vi "Example.vi"   [LabVIEW 2013]
uses:
  T560TriggerClass/T560Trigger.lvclass
  T560SessionClass/T560Session.lvclass
  Common/TypeDefs/TriggerImpedance.ctl
  Common/TypeDefs/ChannelPolarity.ctl
  Common/TypeDefs/TriggerSource.ctl
  T560OutputClass/T560Output.lvclass
  Common/TypeDefs/ChannelName.ctl
  T560ChannelClass/T560Channel.lvclass
types:
  T1 = typedef "T560Channel.lvclass/ChannelName.ctl" = enum16{"Null", "A", "B", "C", "D", "Trigger"}
  T2 = typedef "TriggerSource.ctl" = enum16{"Rising", "Falling", "Internal 80MHz", "Internal DDS", "Remote", "Disabled"}
  T3 = typedef "ChannelPolarity.ctl" = enum16{"Direct", "Inverted"}
  T4 = typedef "TriggerImpedance.ctl" = enum16{"10KOhm", "50Ohms"}
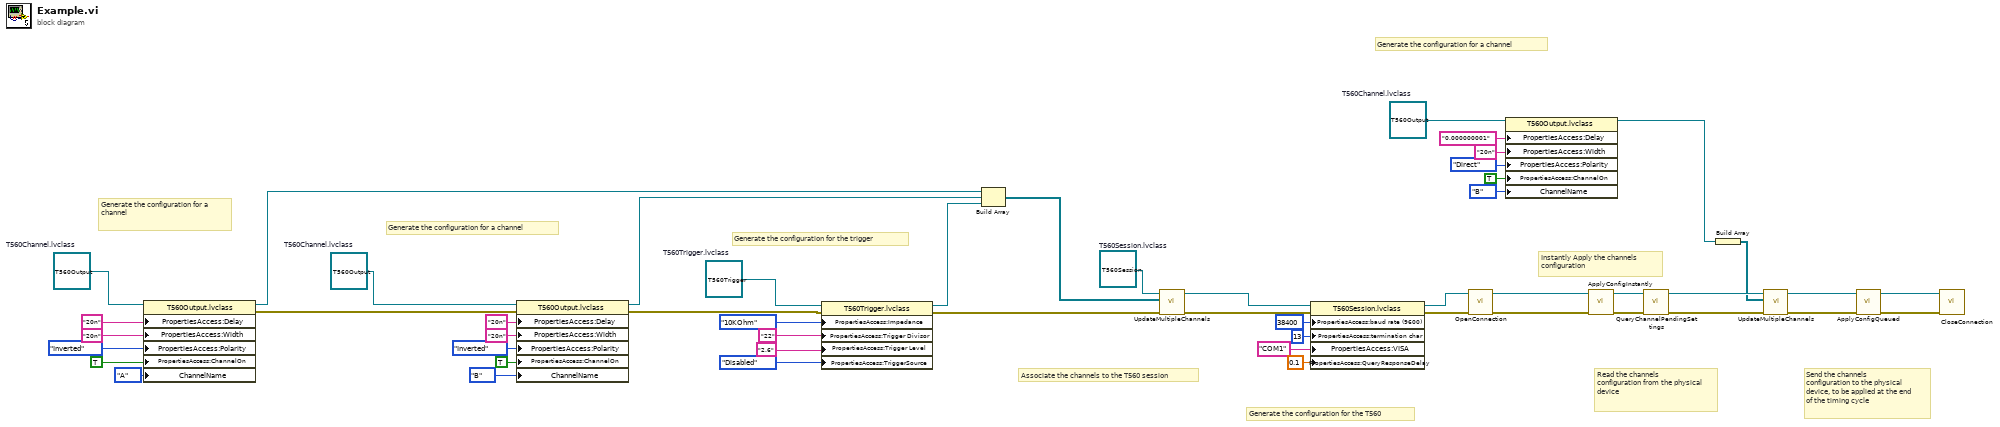
[diagram p0: block diagram]
diagram:
  w21 = refnum<class "T560Output.lvclass"> refnum  # T560Channel.lvclass
  w20 = refnum<class "T560Output.lvclass"> refnum  # T560Channel.lvclass
  w16 = refnum<class "T560Output.lvclass"> refnum  # T560Channel.lvclass
  w10 = refnum<class "T560Session.lvclass"> refnum  # T560Session.lvclass
  w51 = refnum<class "T560Trigger.lvclass"> refnum  # T560Trigger.lvclass
  # "Read the channels configuration from the physical device"
  # "Send the channels configuration to the physical device, to be applied at the end of the timing cycle"
  # "Generate the configuration for a channel"
  # "Instantly Apply the channels \nconfiguration"
  # "Generate the configuration for the T560"
  # "Associate the channels to the T560 session"
  # "Generate the configuration for a channel"
  # "Generate the configuration for the trigger"
  # "Generate the configuration for a channel"
  n1 = property class="T560Output.lvclass"(reference=w16, "PropertiesAccess:Delay"="20n" ("Delay"), "PropertiesAccess:Width"="20n" ("Width"), "PropertiesAccess:Polarity"=ChannelPolarity."Inverted" ("Polarity"), "PropertiesAccess:ChannelOn"=TRUE ("ChannelOn"), "ChannelName"=ChannelName."A") -> (reference out=w36:refnum<class "T560Output.lvclass">, error out=w19:errorcluster)  [unwired: 1 in]
  n2 = property class="T560Output.lvclass"(reference=w20, error in=w19, "PropertiesAccess:Delay"="20n" ("Delay"), "PropertiesAccess:Width"="20n" ("Width"), "PropertiesAccess:Polarity"=ChannelPolarity."Inverted" ("Polarity"), "PropertiesAccess:ChannelOn"=TRUE ("ChannelOn"), "ChannelName"=ChannelName."B") -> (reference out=w35:refnum<class "T560Output.lvclass">, error out=w34:errorcluster)
  n3 = property class="T560Trigger.lvclass"(reference=w51, error in=w34, "PropertiesAccess:Impedance"=TriggerImpedance."10KOhm" ("Impedance"), "PropertiesAccess:Trigger Divisor"="22" ("Trigger Divisor"), "PropertiesAccess:Trigger Level"="2.6" ("Trigger Divisor"), "PropertiesAccess:TriggerSource"=TriggerSource."Disabled" ("TriggerSource")) -> (reference out=w41:refnum<class "T560Trigger.lvclass">, error out=w11:errorcluster)
  n4 = Build Array(w36, w35, w41) -> (w8:refnum<class "T560Channel.lvclass">[])
  n5 = call-dynamic "UpdateMultipleChannels.vi"("error in (no error)"=w11, "ChannelsIn"=w8, "T560Session in"=w10) -> ("error out"=w7:errorcluster, "T560Session out"=w9:refnum<class "T560Session.lvclass">)  [unwired: 7 in]
  n6 = property class="T560Session.lvclass"(reference=w9, error in=w7, "PropertiesAccess:baud rate (9600)"=u32 38400 ("baud rate (9600)"), "PropertiesAccess:termination char"=u8 13 ("termination char"), "PropertiesAccess:VISA"="COM1" ("VISA"), "PropertiesAccess:QueryResponseDelay"=0.1 ("QueryResponseDelay")) -> (reference out=w32:refnum<class "T560Session.lvclass">, error out=w33:errorcluster)
  n7 = call-dynamic "OpenConnection.vi"("error in"=w33, "T560Session in"=w32) -> ("error out"=w43:errorcluster, "T560Session out"=w42:refnum<class "T560Session.lvclass">)  [unwired: 8 in]
  n8 = property class="T560Output.lvclass"(reference=w21, "PropertiesAccess:Delay"="0.000000001" ("Delay"), "PropertiesAccess:Width"="20n" ("Width"), "PropertiesAccess:Polarity"=enum16{"Direct", "Inverted"}."Direct" ("Polarity"), "PropertiesAccess:ChannelOn"=TRUE ("ChannelOn"), "ChannelName"=ChannelName."B") -> (reference out=w5:refnum<class "T560Output.lvclass">)  [unwired: 1 in, 1 out]
  n9 = call-dynamic "ApplyConfigInstantly.vi"("error in"=w43, "T560Session in"=w42) -> ("error out"=w13:errorcluster, "T560Session out"=w14:refnum<class "T560Session.lvclass">)  [unwired: 8 in]
  n10 = call-dynamic "QueryChannelPendingSettings.vi"("error in"=w13, "T560Session in"=w14) -> ("error out"=w3:errorcluster, "T560Session out"=w6:refnum<class "T560Session.lvclass">)  [unwired: 8 in]
  n11 = Build Array(w5) -> (w4:refnum<class "T560Output.lvclass">[])
  n12 = call-dynamic "UpdateMultipleChannels.vi"("error in (no error)"=w3, "ChannelsIn"=w4, "T560Session in"=w6) -> ("error out"=w1:errorcluster, "T560Session out"=w2:refnum<class "T560Session.lvclass">)  [unwired: 7 in]
  n13 = call-dynamic "ApplyConfigQueued.vi"("error in"=w1, "T560Session in"=w2) -> ("error out"=w24:errorcluster, "T560Session out"=w23:refnum<class "T560Session.lvclass">)  [unwired: 8 in]
  n14 = call-dynamic "CloseConnection.vi"("error in"=w24, "T560Session in"=w23) -> ()  [unwired: 8 in, 2 out]
